vi "TextDisplayTester.vi"() -> ()   [LabVIEW 2020]
uses:
  c668da0b-6126-4f41-9ae3-ed63a6a24628.vi
  TextDisplay Class.lvclass
  uiControlsMgr/uiControlsMgr.lvclass
panel:
  out "0009":string
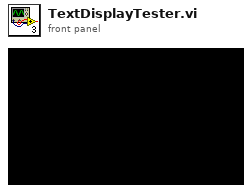
[diagram p1: front panel]
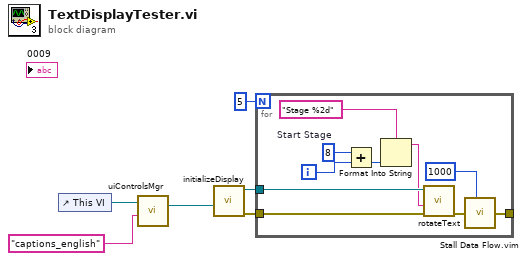
[diagram p0: block diagram]
diagram:
  n1 = control-ref of="This VI"() -> (w3:refnum<vi>)
  n2 = call "uiControlsMgr.vi"("Captions File"="captions_english", "VI reference"=w3) -> ("uiControlsMgr out"=w1:refnum<class "uiControlsMgr.lvclass">)  [unwired: 8 in, 1 out]
  n3 = call "initializeDisplay.vi"("uiControlsMgr.lvclass"=w1) -> ("error out"=w5:errorcluster, "TextDisplay Class out"=w6:refnum<class "TextDisplay Class.lvclass">)  [unwired: 9 in]
  n4 = for {
    N: 5 -> [_]
    tunnel: w6 -> [w16]
    tunnel: w5 -> [w15]
    tunnel: [w10] -> _
    i -> [w14]
    w7 = 8  # Start Stage
    n5 = Add(x=w7, y=w14) -> (x+y=w8:i32)
    n6 = Format Into String(format string="Stage %2d", w8) -> (resulting string=w12:string)  [unwired: 2 in, 1 out]
    n7 = call "rotateText.vi"("error in (no error)"=w15, "textIn"=w12, "TextDisplay Class in"=w16) -> ("error out"=w11:errorcluster)  [unwired: 7 in, 1 out]
    n8 = call "Stall Data Flow.vim"("value in"=w11, "milliseconds to wait"=u32 1000) -> ("value out"=w10:errorcluster)  [unwired: 1 out]
  }
